vi "Format to Display Style.vi"(9 "Format String":string, 11 "error in":errorcluster) -> (2 "Display Style":u32, 3 "error out":errorcluster)   [LabVIEW 2019, in "Quick Format QD.lvlib"]
doc: "Interprets the Format String to give the string Display Style."
uses:
  Quick Format QD.lvlib
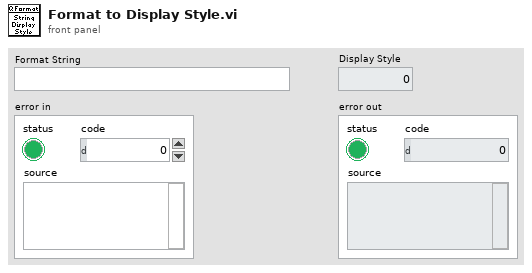
[diagram p1: front panel]
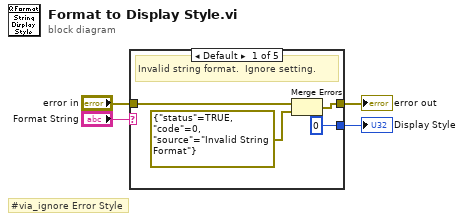
[diagram p0: block diagram]
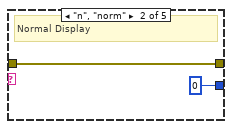
[diagram p2: hidden frame]
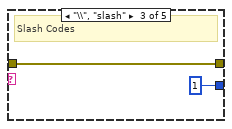
[diagram p3: hidden frame]
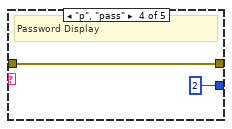
[diagram p4: hidden frame]
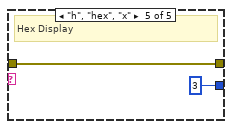
[diagram p5: hidden frame]
diagram:
  # "#via_ignore Error Style"
  n1 = case shown="Default" "Format String" {
    tunnel: "error in" -> [w8 w10 w12 w14 w16]
    tunnel: [w7 w10 w12 w14 w16] -> w3
    tunnel: [u32 0 ("Display Style") u32 0 ("Display Style") u32 1 ("Display Style") u32 2 ("Display Style") u32 3 ("Display Style")] -> w2
    frame Default {
      # "Invalid string format.  Ignore setting."
      n2 = Merge Errors(w8, errorcluster {"status"=TRUE, "code"=0, "source"="Invalid String Format"} ("error constant")) -> (w7:errorcluster)
    }
    frame "n", "norm" {
      # "Normal Display"
    }
    frame "\\", "slash" {
      # "Slash Codes"
    }
    frame "p", "pass" {
      # "Password Display"
    }
    frame "h", "hex", "x" {
      # "Hex Display"
    }
  }
  "Display Style" <- w2
  "error out" <- w3
